vi "logging.vi"(6 "error in (no error)":errorcluster, 9 "Message Queues in":T1) -> (0 "error out":errorcluster)   [LabVIEW 2024]
uses:
  support/Message Queue/All Message Queues.ctl
  support/Message Queue/Message Cluster.ctl
  support/Message Queue/Enqueue Message (Single).vi
  <userlib>/HBM LabVIEW Driver/DLLs/Hbm.Api.Common.dll
  support/Message Queue/Message Queue.lvlib
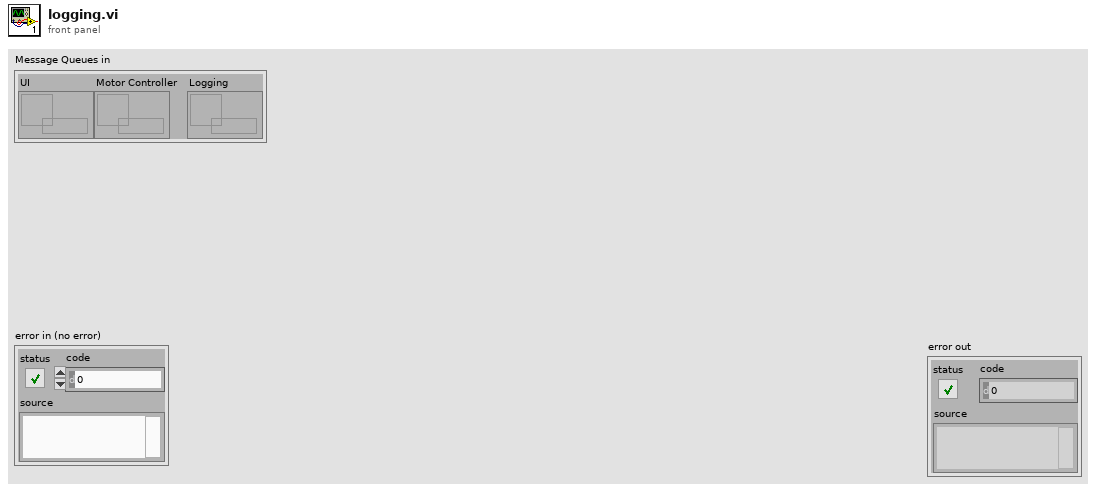
[diagram p1: front panel]
types:
  T1 = typedef "Message Queue.lvlib/All Message Queues.ctl" = cluster{"UI":refnum<queue>, "Motor Controller":refnum<queue>, "Logging":refnum<queue>}
  T2 = cluster{"Devices":refnum<k24>[], "Signals":refnum<k24>[]}
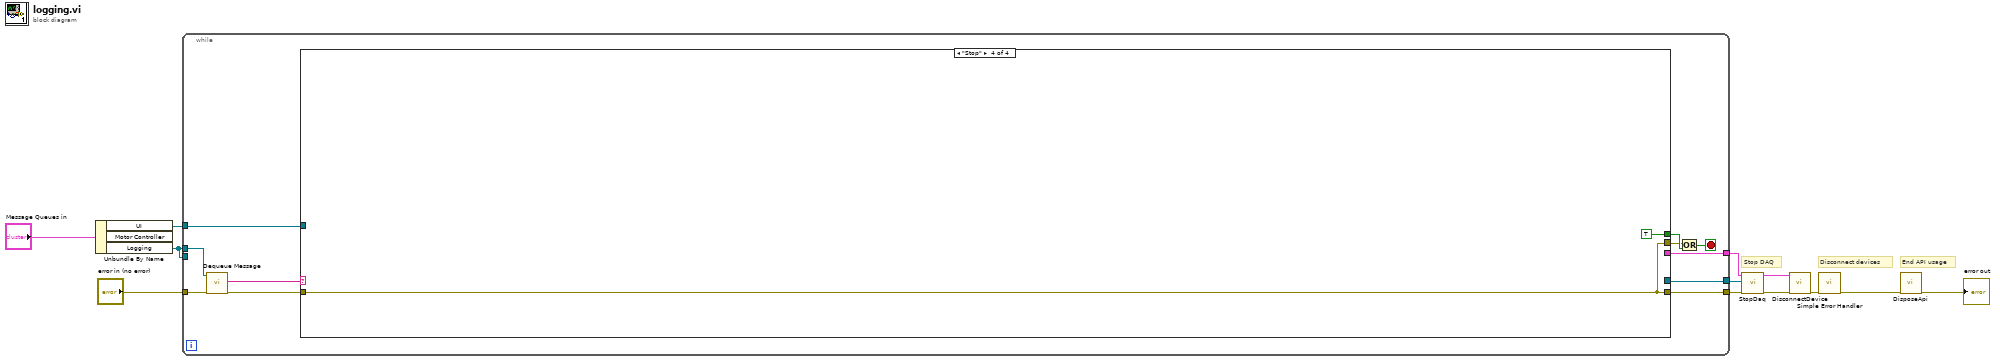
[diagram p0: block diagram]
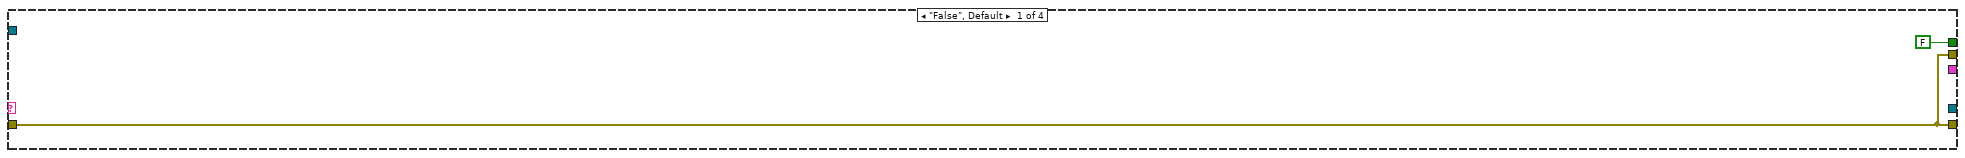
[diagram p2: hidden frame]
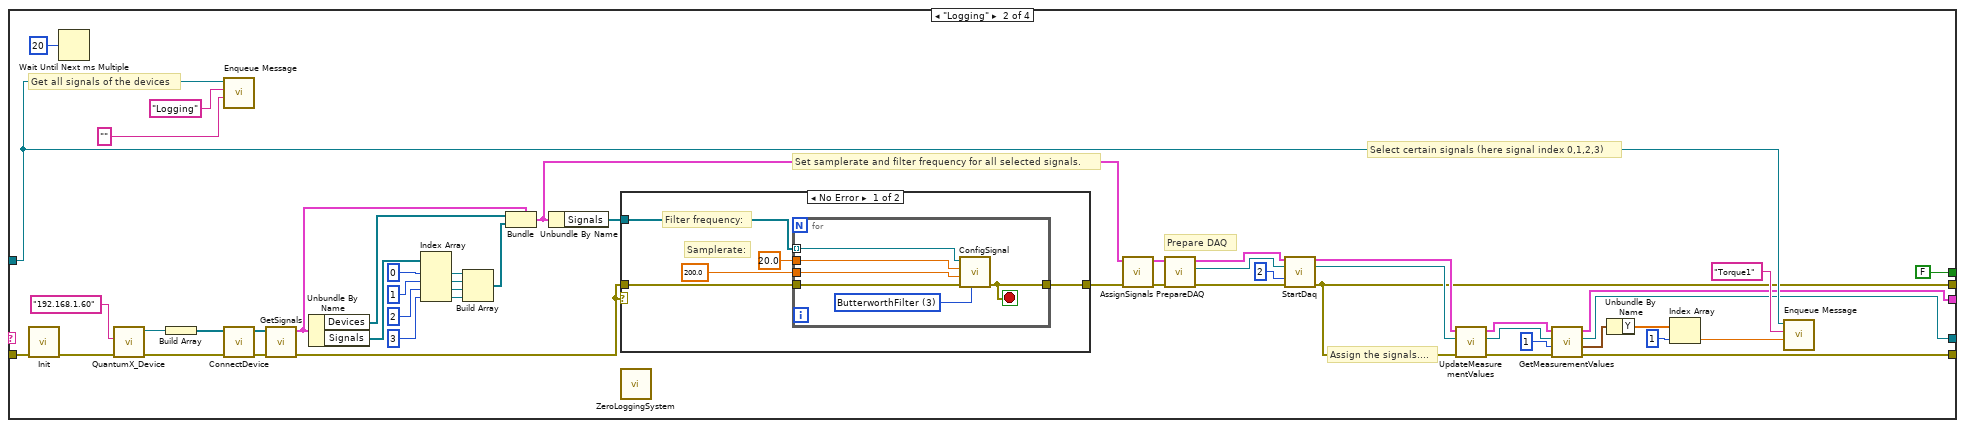
[diagram p3: hidden frame]
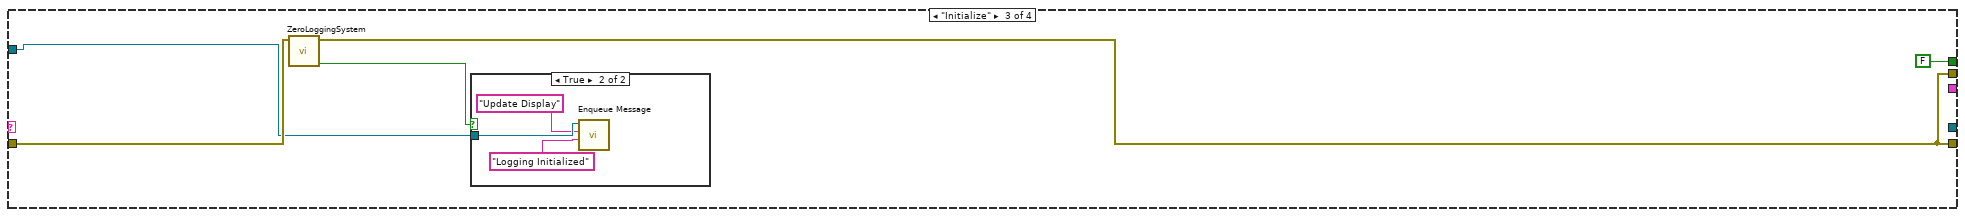
[diagram p5: hidden frame]
diagram:
  # "Disconnect devices"
  # "End API usage"
  # "Stop DAQ"
  n1 = Unbundle By Name("Message Queues in") -> ("UI"=w11:refnum<queue>, "Logging"=w10:refnum<queue>)  [unwired: 1 out]
  n2 = while {
    tunnel: w10 -> [w23]
    tunnel: w11 -> [w16]
    tunnel: w10 -> [_]
    tunnel: [w15] -> w5
    tunnel: [w14] -> w4
    tunnel: [w19] -> w3
    tunnel: "error in (no error)" -> [w18]
    stop <- w21 stop-if-true
    n3 = call "Dequeue Message.vi"("error in (no error)"=w18, "Message Queue"=w23) -> ("error out"=w17:errorcluster, "Message"=w22:string)  [unwired: 6 in, 2 out]
    n4 = case shown="\"Stop\"" w22 {
      tunnel: [FALSE FALSE FALSE TRUE] -> w20
      tunnel: [w24 w26 w90 w96] -> w19
      tunnel: w17 -> [w24 w46 w91 w96]
      tunnel: w16 -> [_ w32 w88 _]
      tunnel: [_ w29 _ _] -> w15
      tunnel: [_ w28 _ _] -> w14
      tunnel: [w24 w27 w90 w96] -> w13
      frame "False", Default {
      }
      frame "Logging" {
        # "Set samplerate and filter frequency for all selected signals."
        # "Prepare DAQ"
        # "Select certain signals (here signal index 0,1,2,3)"
        # "Get all signals of the devices"
        # "Assign the signals...."
        n5 = call <userlib>:"Init.vi"("Error in"=w46) -> ("Error out"=w52:errorcluster)  [unwired: 7 in, 2 out]
        n6 = Wait Until Next ms Multiple(millisecond multiple=u32 20 ("Vielfache von ms")) -> ()  [unwired: 1 out]
        n7 = call <userlib>:"QuantumX_Device.vi"("Error in"=w52, "IPAddress"="192.168.1.60" ("IPAddress of QuantumX device")) -> ("Error out"=w53:errorcluster, "Device"=w50:refnum<k24>)  [unwired: 6 in]
        n8 = Build Array(w50) -> (w49:refnum<k24>[])
        n9 = call-poly "Enqueue Message.vi"("Message Data"="", "Message"="Logging", "Message Queue"=w32) -> ()  [unwired: 7 in, 2 out]
        n10 = call <userlib>:"ConnectDevice.vi"("Error in"=w53, "Devices"=w49) -> ("Error out"=w68:errorcluster, "Devices"=w67:refnum<k24>[])  [unwired: 7 in, 1 out]
        n11 = call <userlib>:"GetSignals.vi"("Error in"=w68, "Devices"=w67) -> ("Error out"=w47:errorcluster, "DevicesAndSignals"=w48:T2)  [unwired: 8 in]
        n12 = Unbundle By Name(w48) -> ("Devices"=w60:refnum<k24>[], "Signals"=w64:refnum<k24>[])
        n13 = Index Array(array=w64, index #1=0 ("Index"), index #2=1 ("Index"), index #3=2 ("Index"), index #4=3 ("Index")) -> (element #1=w63:refnum<k24>, element #2=w62:refnum<k24>, element #3=w55:refnum<k24>, element #4=w54:refnum<k24>)
        n14 = Build Array(w63, w62, w55, w54) -> (w61:refnum<k24>[])
        n15 = Bundle(cluster=w48, "Devices"=w60, "Signals"=w61) -> (w66:T2)
        n16 = Unbundle By Name(w66) -> ("Signals"=w75:refnum<k24>[])
        n17 = case shown="No Error" w47 {
          tunnel: w47 -> [w80 w87]
          tunnel: w75 -> [w79 _]
          tunnel: [w78 w87] -> w74
          frame No Error {
            # "Filter frequency:"
            # "Samplerate:"
            n18 = for {
              tunnel: w80 -> [w86]
              tunnel: 200.0 ("SampleRate") -> [w85]
              tunnel: 20.0 ("FilterFrequency") -> [w84]
              tunnel: w79 -> [w83] mode=indexing
              tunnel: [w82] -> w78
              stop <- w82 stop-if-true
              w81 = 3 items=["PresentFilter", "AutoFilter", "BesselFilter", "ButterworthFilter", "HighpassFilter", "LinearPhaseFilter", "NoFilter"] ("FilterType")
              n19 = call <userlib>:"ConfigSignal.vi"("FilterType"=w81, "Error in"=w86, "SampleRate"=w85, "FilterFrequency"=w84, "Signal"=w83) -> ("Error out"=w82:errorcluster)  [unwired: 6 in]
            }
          }
          frame Error {
          }
        }
        n20 = call "ZeroLoggingSystem.vi"() -> ()  [unwired: 10 in, 2 out]
        n21 = call <userlib>:"AssignSignals.vi"("Error in"=w74, "DevicesAndSignals"=w66) -> ("Error out"=w72:errorcluster, "DevicesAndSignals"=w73:T2)  [unwired: 8 in]
        n22 = call <userlib>:"PrepareDAQ.vi"("Error in"=w72, "DevicesAndSignals"=w73) -> ("Error out"=w69:errorcluster, "DaqMeasurement"=w70:refnum<k24>, "DevicesAndSignals"=w71:T2)  [unwired: 7 in]
        n23 = call <userlib>:"StartDaq.vi"("DevicesAndSignals"=w71, "DaqMeasurement"=w70, "AcquisitionMode"=2, "Error in"=w69) -> ("DevicesAndSignals"=w31:T2, "DaqMeasurement"=w30:refnum<k24>, "Error out"=w27:errorcluster)  [unwired: 7 in, 2 out]
        n24 = call <userlib>:"UpdateMeasurementValues.vi"("Error in"=w27, "DaqMeasurement"=w30, "DevicesAndSignals"=w31) -> ("Error out"=w40:errorcluster, "DaqMeasurement"=w41:refnum<k24>, "DevicesAndSignals"=w42:T2)  [unwired: 6 in]
        n25 = call <userlib>:"GetMeasurementValues.vi"("Error in"=w40, "Index"=1 ("Signal index to display"), "DaqMeasurement"=w41, "DevicesAndSignals"=w42) -> ("Error out"=w26:errorcluster, "Waveform"=w37:waveform(dbl), "DaqMeasurement"=w28:refnum<k24>, "DevicesAndSignals"=w29:T2)  [unwired: 2 in, 2 out]
        n26 = Unbundle By Name(w37) -> ("Y"=w36:dbl[])
        n27 = Index Array(array=w36, index=1) -> (element=w33:dbl)
        n28 = call-poly "Enqueue Message.vi"("Message Data"=w33, "Message"="Torque1", "Message Queue"=w32) -> ()  [unwired: 7 in, 2 out]
      }
      frame "Initialize" {
        n29 = call "ZeroLoggingSystem.vi"("Error in"=w91) -> ("Complete"=w89:bool, "Error out"=w90:errorcluster)  [unwired: 9 in]
        n30 = case shown="True" w89 {
          tunnel: w88 -> [_ w95]
          frame False {
          }
          frame True {
            n31 = call-poly "Enqueue Message.vi"("Message Data"="Logging Initialized", "Message"="Update Display", "Message Queue"=w95) -> ()  [unwired: 7 in, 2 out]
          }
        }
      }
      frame "Stop" {
      }
    }
    n32 = Or(x=w13, y=w20) -> (x .or. y?=w21:bool)
  }
  n33 = call <userlib>:"StopDaq.vi"("Error in"=w3, "DaqMeasurement"=w4, "DevicesAndSignals"=w5) -> ("Error out"=w8:errorcluster, "DevicesAndSignals"=w7:T2)  [unwired: 7 in]
  n34 = call <userlib>:"DisconnectDevice.vi"("Error in"=w8, "DevicesAndSignals"=w7) -> ("Error out"=w6:errorcluster)  [unwired: 9 in]
  n35 = call <vilib>:"Simple Error Handler.vi"("error in (no error)"=w6) -> ("error out"=w9:errorcluster)  [unwired: 4 in, 4 out]
  n36 = call <userlib>:"DisposeApi.vi"("Error in"=w9) -> ("Error out"=→"error out":errorcluster)  [unwired: 10 in]
